vi "pythagoras.vi"(1 "b":dbl, 2 "a":dbl) -> (0 "c":dbl)   [LabVIEW 2020, in "POLARIS Vision utility.lvlib"]
uses:
  POLARIS Vision utility.lvlib
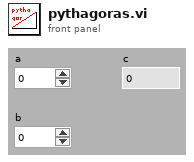
[diagram p1: front panel]
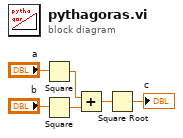
[diagram p0: block diagram]
diagram:
  n1 = Square(x="a") -> (x^2=w1:dbl)
  n2 = Square(x="b") -> (x^2=w3:dbl)
  n3 = Add(x=w1, y=w3) -> (x+y=w2:dbl)
  n4 = Square Root(x=w2) -> (sqrt(x)=→"c":dbl)
